vi "CRYPEAQ Harmonic Struct Error.vi"(0 "Level Adaptation -> EarWeighted Stimulus":dbl[](array[numeric]), 1 "Stimulus":dbl[](array[numeric]), 2 "Correlation Point Number":dbl=2048.0, 3 "Response":dbl[](array[numeric]), 5 "EarWeighted Response":dbl[](array[numeric]), 7 "Fc Hz":dbl, 12 "Fs":dbl=44100.0, 13 "Hanning Window":dbl[](array[numeric]), 14 "NF":dbl=2048.0) -> (6 "EHS":dbl)   [LabVIEW 2013]
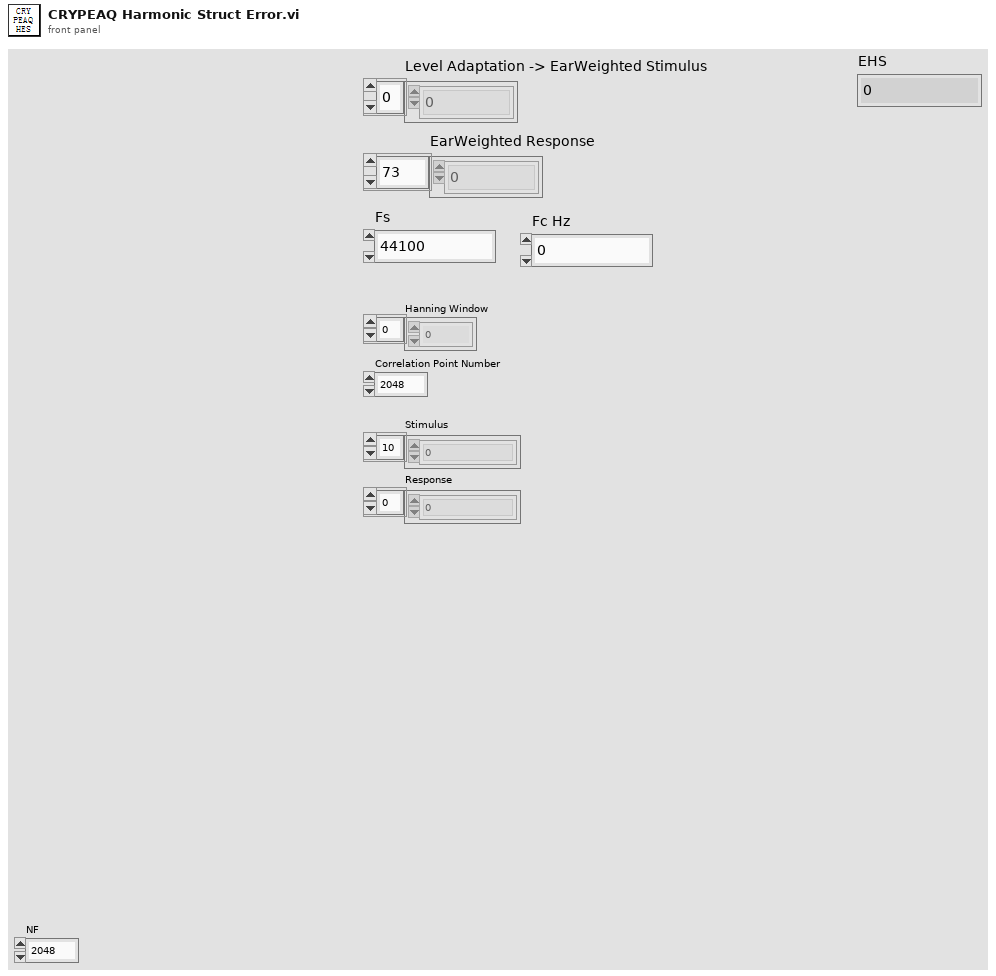
[diagram p1: front panel]
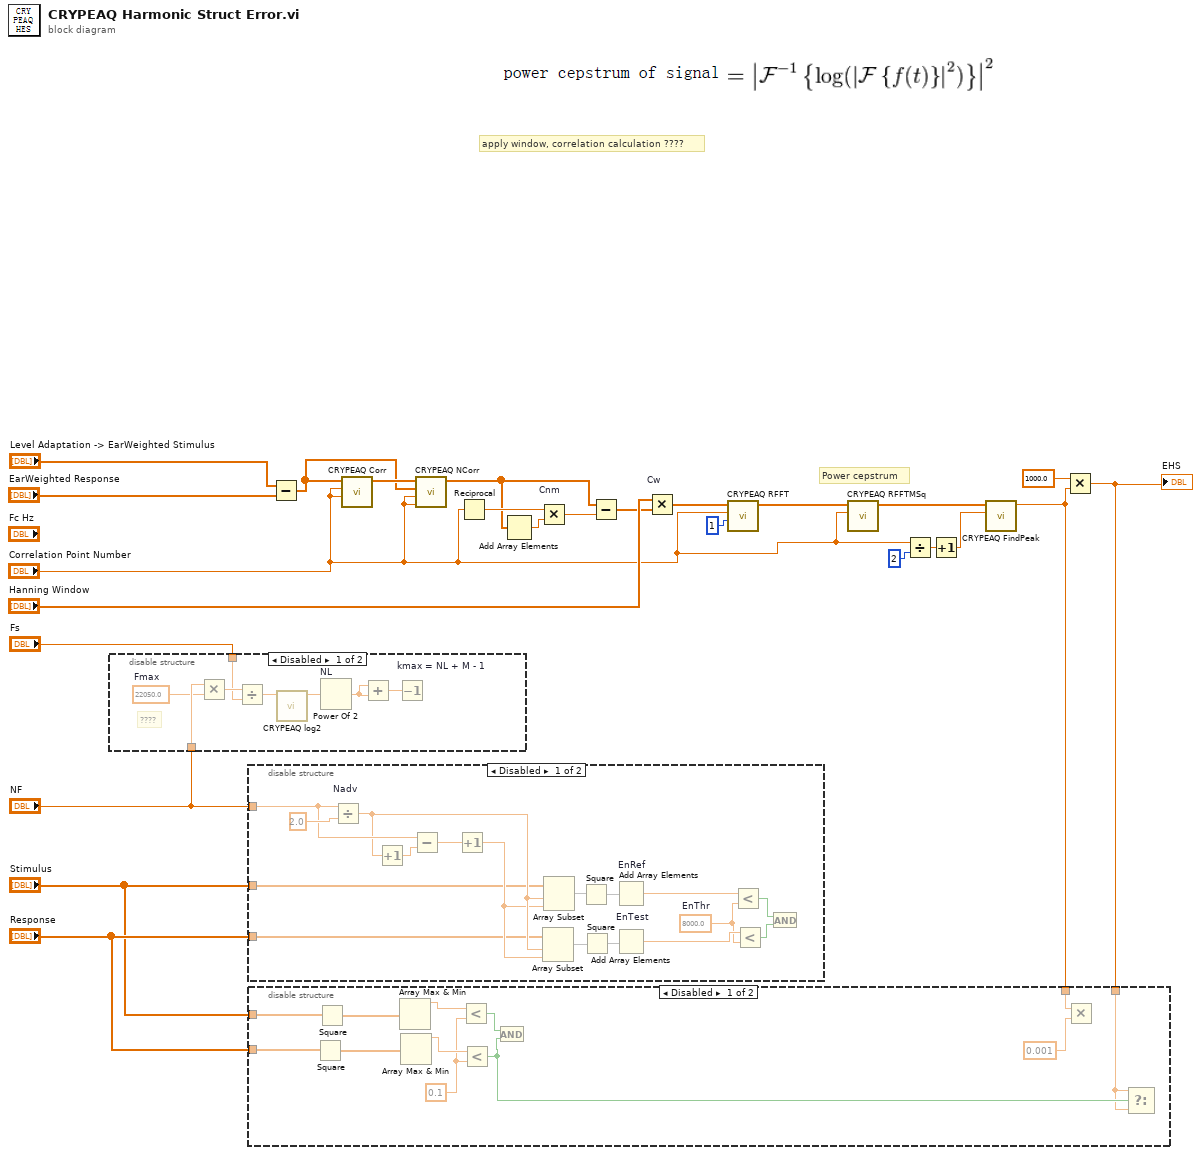
[diagram p0: block diagram]
diagram:
  # "Power cepstrum"
  # "apply window, correlation calculation ????"
  n1 = disable-structure shown="Disabled" {
    disable-tunnel: "NF" -> [w31 _]
    disable-tunnel: "Fs" -> [w27 _]
    frame Disabled {
      w26 = 22050.0  # Fmax
      # "????"
      n2 = Multiply(x=w31, y=w26) -> (x*y=w30:dbl)
      n3 = Divide(x=w30, y=w27) -> (x/y=w29:dbl)
      n4 = call "CRYPEAQ log2.vi"("a"=w29) -> ("log2"=w32:dbl)  [unwired: 10 in]
      n5 = Power Of 2 "NL"(x=w32) -> (2^x=w28:dbl)
      n6 = Add(x=w28, y=w28) -> (x+y=w33:dbl)
      n7 = Decrement "kmax = NL + M - 1"(x=w33) -> ()  [unwired: 1 out]
    }
    frame Enabled {
    }
  }
  n8 = disable-structure shown="Disabled" {
    disable-tunnel: "NF" -> [w49 _]
    disable-tunnel: "Response" -> [w35 _]
    disable-tunnel: "Stimulus" -> [w34 _]
    frame Disabled {
      w36 = 8000.0  # EnThr
      n9 = Divide "Nadv"(x=w49, y=2.0) -> (x/y=w48:dbl)
      n10 = Increment(x=w48) -> (x+1=w39:dbl)
      n11 = Subtract(x=w49, y=w39) -> (x-y=w38:dbl)
      n12 = Increment(x=w38) -> (x+1=w37:dbl)
      n13 = Array Subset(array=w35, index=w48, length=w37) -> (w46:dbl[])
      n14 = Array Subset(array=w34, index=w48, length=w37) -> (w47:dbl[])
      n15 = Square(x=w47) -> (x^2=w45:dbl[])
      n16 = Square(x=w46) -> (x^2=w44:dbl[])
      n17 = Add Array Elements "EnRef"(numeric array=w45) -> (sum=w43:dbl)
      n18 = Add Array Elements "EnTest"(numeric array=w44) -> (sum=w42:dbl)
      n19 = Less?(x=w43, y=w36) -> (x < y?=w41:bool)
      n20 = Less?(x=w42, y=w36) -> (x < y?=w40:bool)
      n21 = And(x=w41, y=w40) -> ()  [unwired: 1 out]
    }
    frame Enabled {
    }
  }
  n22 = Subtract(x="Level Adaptation -> EarWeighted Stimulus", y="EarWeighted Response") -> (x-y=w5:dbl[])
  n23 = call "CRYPEAQ Corr.vi"("M"="Correlation Point Number", "NL"="Correlation Point Number", "D"=w5) -> ("C"=w14:dbl[])  [unwired: 8 in]
  n24 = call "CRYPEAQ NCorr.vi"("M"="Correlation Point Number", "NL"="Correlation Point Number", "D"=w5, "C"=w14) -> ("Cn"=w9:dbl[])  [unwired: 7 in]
  n25 = Reciprocal(x="Correlation Point Number") -> (1/x=w17:dbl)
  n26 = Add Array Elements(numeric array=w9) -> (sum=w18:dbl)
  n27 = Multiply "Cnm"(x=w17, y=w18) -> (x*y=w16:dbl)
  n28 = Subtract(x=w9, y=w16) -> (x-y=w8:dbl[])
  n29 = Multiply "Cw"(x="Hanning Window", y=w8) -> (x*y=w7:dbl[])
  n30 = call "CRYPEAQ RFFT.vi"("ifn"=1, "N"="Correlation Point Number", "x"=w7) -> ("X"=w6:dbl[])  [unwired: 8 in]
  n31 = call "CRYPEAQ RFFTMSq.vi"("N"="Correlation Point Number", "X"=w6) -> ("X2"=w4:dbl[])  [unwired: 9 in]
  n32 = Divide(x="Correlation Point Number", y=2) -> (x/y=w12:dbl)
  n33 = Increment(x=w12) -> (x+1=w11:dbl)
  n34 = call "CRYPEAQ FindPeak.vi"("N"=w11, "c2"=w4) -> ("cmax(EHS)"=w3:dbl)  [unwired: 8 in, 1 out]
  n35 = Multiply(x=1000.0 ("y"), y=w3) -> (x*y=w2:dbl)
  "EHS" <- w2
  n36 = disable-structure shown="Disabled" {
    disable-tunnel: "Response" -> [w62 _]
    disable-tunnel: "Stimulus" -> [w59 _]
    disable-tunnel: w3 -> [w53 _]
    disable-tunnel: w2 -> [w51 _]
    frame Disabled {
      w54 = 0.1 ("y")
      n37 = Square(x=w62) -> (x^2=w61:dbl[])
      n38 = Square(x=w59) -> (x^2=w58:dbl[])
      n39 = Array Max & Min(array=w58) -> (max value=w57:dbl)  [unwired: 3 out]
      n40 = Array Max & Min(array=w61) -> (max value=w60:dbl)  [unwired: 3 out]
      n41 = Less?(x=w57, y=w54) -> (x < y?=w56:bool)
      n42 = Less?(x=w60, y=w54) -> (x < y?=w55:bool)
      n43 = And(x=w56, y=w55) -> ()  [unwired: 1 out]
      n44 = Multiply(x=w53, y=0.001) -> ()  [unwired: 1 out]
      n45 = Select(t=w51, s=w55, f=w51) -> ()  [unwired: 1 out]
    }
    frame Enabled {
    }
  }
